vi "FPGA_SPI_ConfigureAuto.vi"(0 "SPI Bus":T1, 1 "SPI Auto TX Byte Array":u8[](array[numeric]), 2 "SPI Auto TX Zero Byte Array":u8[](array[numeric]), 3 "error in":errorcluster) -> (10 "error out":errorcluster)   [LabVIEW 2017]
uses:
  <vilib>/Rock Robotics/SystemInterfaces/spilib/spi_bus.ctl
  <vilib>/Utility/error.llb/Error Cluster From Error Code.vi
  <vilib>/rvi/errors/niLvFpgaAdjustHostInterfaceError.vi
  <vilib>/rvi/interface/nirviMethod/nirviMethod.xnode
  <vilib>/Rock Robotics/SystemInterfaces/System/FPGA_SystemFRC FPGA Ref.ctl
  <vilib>/rvi/interface/nirviReadWriteControl/nirviReadWriteControl.xnode
  <vilib>/FPGAPlugInAG/Dynamic/niLvFpga_StartFifo_Dynamic.vi
  <vilib>/rvi/errors/niLvFpgaMergeErrorWithErrorCode.vi
  NiFpgaLv.dll
  <vilib>/rvi/interface/Simulation/niFpgaSimulationCallBeginRW.vi
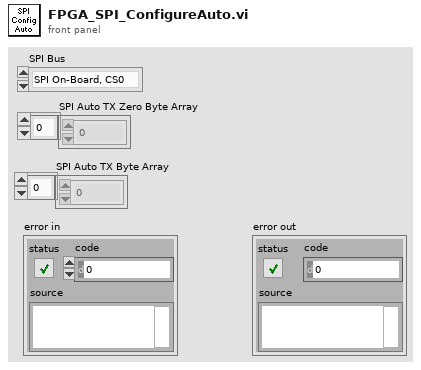
[diagram p1: front panel]
types:
  T1 = typedef "spi_bus.ctl" = enum16{"SPI On-Board, CS0", "SPI On-Board, CS1", "SPI On-Board, CS2", "SPI On-Board, CS3", "SPI MXP", "Invalid"}
  T2 = cluster{"TxByteCount":fxp<+,4,4>, "ZeroByteCount":fxp<+,7,7>}
  T3 = typedef "FPGA_SystemFRC FPGA Ref.ctl" = refnum<k20>
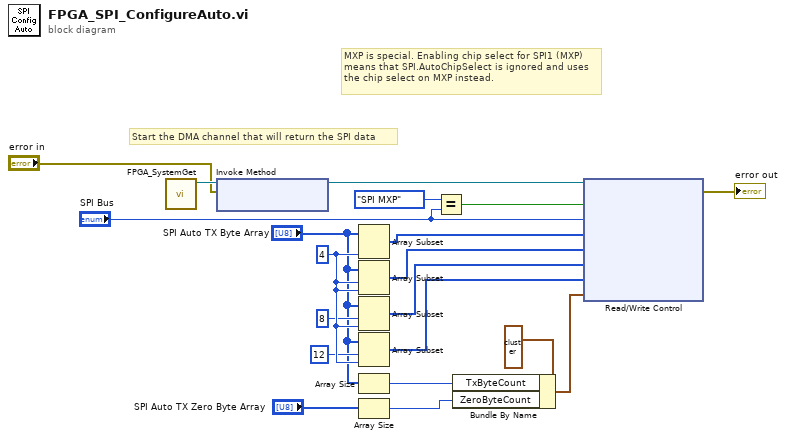
[diagram p0: block diagram]
diagram:
  w13 = 4 ("length")
  # "MXP is special. Enabling chip select for SPI1 (MXP) means that SPI.AutoChipSelect is ignored and uses the chip select on MXP instead."
  # "Start the DMA channel that will return the SPI data"
  n1 = call <vilib>:"FPGA_SystemGet.vi"() -> ("FRC FPGA Ref"=w19:T3)  [unwired: 11 in]
  n2 = xnode "Invoke Method"("FPGA VI Reference In"=w19, "error in"="error in") -> ("FPGA VI Reference Out"=w20:T3)  [unwired: 1 out]
  n3 = Array Subset(array="SPI Auto TX Byte Array", length=w13) -> (w8:u8[])  [unwired: 1 in]
  n4 = Array Subset(array="SPI Auto TX Byte Array", index=w13, length=w13) -> (w7:u8[])
  n5 = Array Subset(array="SPI Auto TX Byte Array", index=8, length=w13) -> (w6:u8[])
  n6 = Array Subset(array="SPI Auto TX Byte Array", index=12, length=w13) -> (w5:u8[])
  n7 = Array Size(array="SPI Auto TX Byte Array") -> (size(s)=w15:i32)
  n8 = Array Size(array="SPI Auto TX Zero Byte Array") -> (size(s)=w1:i32)
  n9 = Equal?(x=spi_bus."SPI MXP", y="SPI Bus") -> (x = y?=w16:bool)
  n10 = Bundle By Name(cluster=T2 {"TxByteCount"=0.0, "ZeroByteCount"=0.0} ("SPI.AutoByteCount"), "TxByteCount"=w15, "ZeroByteCount"=w1) -> (w3:T2)
  n11 = xnode "Read/Write Control"("FPGA VI Reference In"=w20, "SPI.AutoSPI1Select"=w16, "SPI.AutoChipSelect"="SPI Bus", "SPI.AutoTx0"=w8, "SPI.AutoTx1"=w7, "SPI.AutoTx2"=w6, "SPI.AutoTx3"=w5, "SPI.AutoByteCount"=w3) -> ("error out"=→"error out":errorcluster)  [unwired: 1 in, 1 out]
